vi "Test Actions.vi"(6 "data in":T2, 11 "Action":T3) -> (0 "error out":errorcluster, 2 "events out":T1[](array[typedef]), 4 "data out":T2)   [LabVIEW 2019, in "ANODE Tests.lvlib" / "State Machine API.lvlib"]
uses:
  State Machine API.lvlib
  types/Data.ctl
  types/Action.ctl
  types/Event.ctl
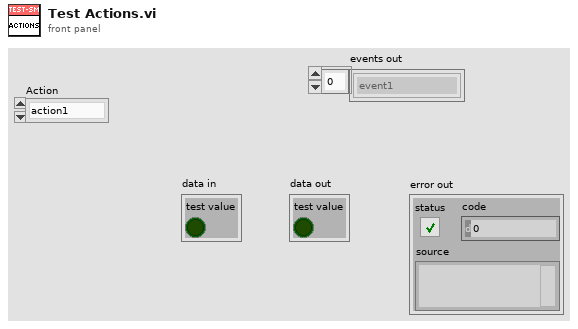
[diagram p1: front panel]
types:
  T1 = typedef "ANODE Tests.lvlib/State Machine API.lvlib/Event.ctl" = enum16{"event1", "event2", "event3"}
  T2 = typedef "ANODE Tests.lvlib/State Machine API.lvlib/Data.ctl" = cluster{"test value":bool}
  T3 = typedef "ANODE Tests.lvlib/State Machine API.lvlib/Action.ctl" = enum16{"action1"}
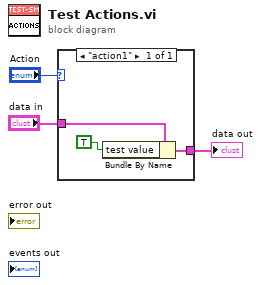
[diagram p0: block diagram]
diagram:
  n1 = case shown="\"action1\"" "Action" {
    tunnel: "data in" -> [w6]
    tunnel: [w5] -> w1
    frame "action1" {
      n2 = Bundle By Name(cluster=w6, "test value"=TRUE) -> (w5:T2)
    }
  }
  "data out" <- w1
